vi "execution class name.vi"(8 "error in":errorcluster, 11 "dds configuration in":refnum<class "dds configuration.lvclass">) -> (0 "error out":errorcluster, 2 "class name":string, 3 "dds configuration out":refnum<class "dds configuration.lvclass">)   [LabVIEW 2020, in "DDS configuration.lvclass"]
doc: "Provides an interface for determining the module runtime class associated with this module configuration. This class name can then be used to dynamically load or locate the runtime class for initialization purposes."
uses:
  dds configuration.lvclass
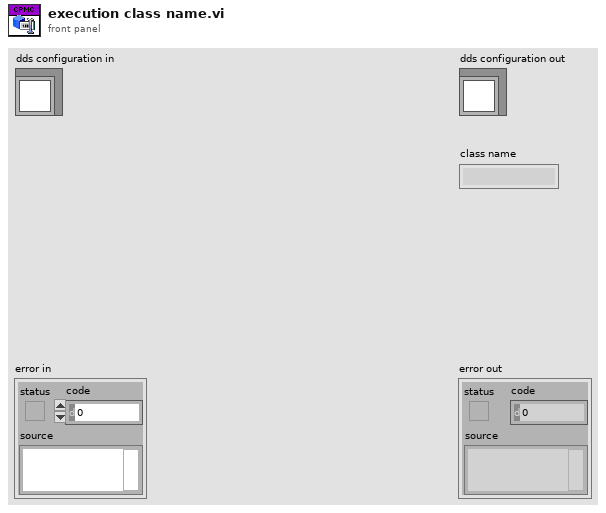
[diagram p1: front panel]
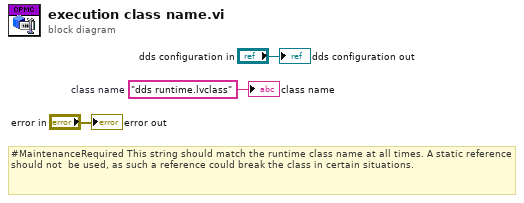
[diagram p0: block diagram]
diagram:
  w1 = "dds runtime.lvclass"  # class name
  # "#MaintenanceRequired This string should match the runtime class name at all times. A static reference should not  be used, as such a reference could break the class in certain situations."
  "error out" <- "error in"
  "dds configuration out" <- "dds configuration in"
  "class name" <- w1
